vi "Initialize.vi"(8 "error in":errorcluster, 11 "Plugin in":refnum<class "Stereo Microphone Input.lvclass">) -> (0 "error out":errorcluster, 3 "Plugin out":refnum<class "Stereo Microphone Input.lvclass">)   [LabVIEW 2026, in "Stereo Microphone Input.lvlib" / "Stereo Microphone Input.lvclass"]
uses:
  Stereo Microphone Input.lvclass
  C:/Program Files/National Instruments/LabVIEW 2026/vi.lib/FlexLogger/SDK/PluginSDK.lvlibp/PEFClasses/SDK/Plugin/Plugin.lvclass
  <vilib>/FlexLogger/SDK/PluginSDK.lvlibp/PEFClasses/SDK/Processing Element/Timing Parameters.ctl
  <vilib>/FlexLogger/SDK/PluginSDK.lvlibp/PEFClasses/SDK/Processing Element/Timing Method.ctl
  <vilib>/FlexLogger/SDK/PluginSDK.lvlibp/PEFClasses/SDK/Producer Channel/Producer Channel.lvclass
  C:/Program Files/National Instruments/LabVIEW 2026/vi.lib/FlexLogger/SDK/PluginSDK.lvlibp/PEFClasses/SDK/Channel/Channel.lvclass
  <vilib>/FlexLogger/SDK/PluginSDK.lvlibp/PEFClasses/SDK/Plugin/ParameterAccess/Write String.vi
  <vilib>/FlexLogger/SDK/PluginSDK.lvlibp/PEFClasses/SDK/Plugin/ParameterAccess/Write DBL.vi
  <vilib>/FlexLogger/SDK/PluginSDK.lvlibp/PEFClasses/SDK/Producer Channel/Create Producer Channel_v2.vi
  <vilib>/FlexLogger/SDK/PluginSDK.lvlibp/PEFClasses/SDK/Channel/ParameterAccess/Write DBL.vi
  <vilib>/FlexLogger/SDK/PluginSDK.lvlibp/PEFClasses/SDK/Plugin/Plugin.lvclass
  C:/Program Files/National Instruments/LabVIEW 2026/vi.lib/FlexLogger/SDK/PluginSDK.lvlibp/PEFClasses/SDK/Processing Element/Processing Element.lvclass
  C:/Users/nkirchne/Documents/LabVIEW Projects/FlexLogger IO Plug-ins/Stereo Microphone Input/Stereo Microphone Input.lvclass
  C:/Program Files/National Instruments/LabVIEW 2026/vi.lib/FlexLogger/SDK/PluginSDK.lvlibp/PEFClasses/SDK/Producer Channel/Producer Channel.lvclass
  <vilib>/FlexLogger/SDK/PluginSDK.lvlibp/PEFClasses/SDK/Processing Element/Processing Element.lvclass
  <vilib>/FlexLogger/SDK/PluginSDK.lvlibp/PEFClasses/SDK/Channel/Channel.lvclass
  <vilib>/FlexLogger/SDK/PluginSDK.lvlibp
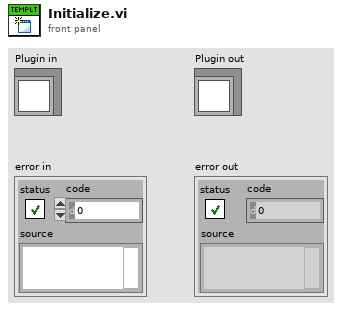
[diagram p1: front panel]
types:
  T1 = typedef "PluginSDK.lvlibp/Processing Element.lvclass/Timing Parameters.ctl" = cluster{"Timing Method":T2, "Timing Period (ms)":i32}
  T2 = typedef "PluginSDK.lvlibp/Processing Element.lvclass/Timing Method.ctl" = enum16{"Periodic", "Immediate", "On Data Ready", "Triggered"}
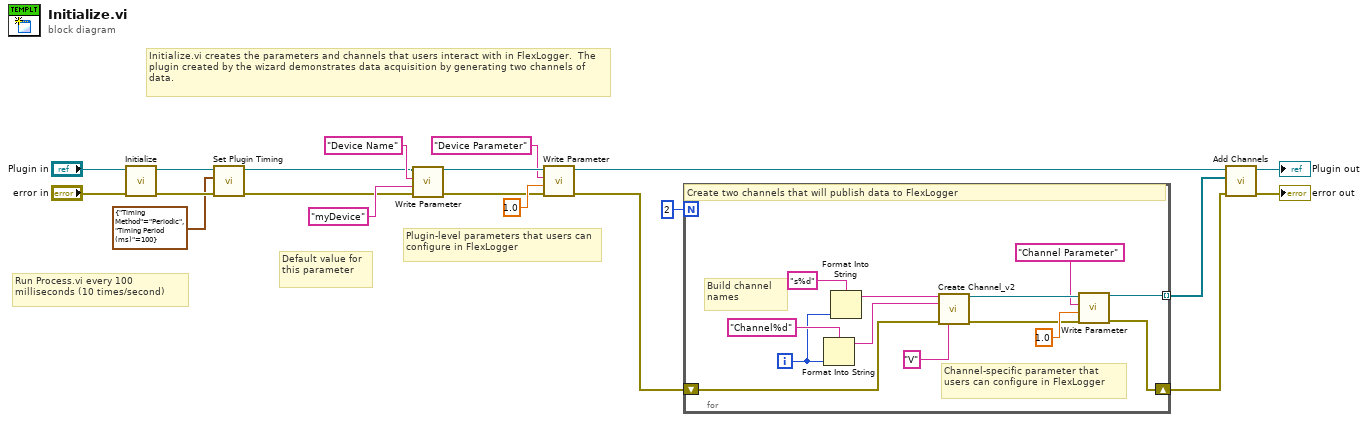
[diagram p0: block diagram]
diagram:
  # "Default value for this parameter"
  # "Plugin-level parameters that users can configure in FlexLogger"
  # "Run Process.vi every 100 milliseconds (10 times/second)"
  # "Initialize.vi creates the parameters and channels that users interact with in FlexLogger.  The plugin created by the wizard demonstrates data acquisition by generating two channels of data."
  n1 = call-parent "Initialize.vi"("error in (no error)"="error in", "Plugin in"="Plugin in") -> ("error out"=w5:errorcluster, "Plugin out"=w3:refnum<class "Stereo Microphone Input.lvclass">)  [unwired: 8 in]
  n2 = call <vilib>:"Set Plugin Timing.vi"("error in (no error)"=w5, "Timing Parameters"=T1 {"Timing Method"=enum."Periodic", "Timing Period (ms)"=100}, "Plugin in"=w3) -> ("error out"=w1:errorcluster, "Plugin out"=w2:refnum<class "Stereo Microphone Input.lvclass">)  [unwired: 7 in]
  n3 = call-poly <vilib>:"Write Parameter.vi"("error in (no error)"=w1, "Value"="myDevice", "Name"="Device Name", "Plugin in"=w2) -> ("error out"=w9:errorcluster, "Plugin out"=w14:refnum<class "Stereo Microphone Input.lvclass">)  [unwired: 6 in]
  n4 = call-poly <vilib>:"Write Parameter.vi"("error in (no error)"=w9, "Value"=1.0, "Name"="Device Parameter", "Plugin in"=w14) -> ("error out"=w8:errorcluster, "Plugin out"=w13:refnum<class "Stereo Microphone Input.lvclass">)  [unwired: 6 in]
  n5 = for {
    N: 2 -> [_]
    shift-right: [w23] -> w15
    shift-left: w8 -> [w22]
    tunnel: [w25] -> w7 mode=indexing
    i -> [w24]
    # "Build channel names"
    # "Channel-specific parameter that users can configure in FlexLogger"
    # "Create two channels that will publish data to FlexLogger"
    n6 = Format Into String(format string="Channel%d", w24) -> (resulting string=w32:string)  [unwired: 2 in, 1 out]
    n7 = Format Into String(format string="s%d", w24) -> (resulting string=w31:string)  [unwired: 2 in, 1 out]
    n8 = call-poly <vilib>:"Create Channel_v2.vi"("Unique Channel Identifier"=w31, "Default Channel Name"=w32, "error in (no error)"=w22, "Unit"="V") -> ("Producer Channel"=w33:refnum<class "Producer Channel.lvclass">, "error out"=w21:errorcluster)  [unwired: 10 in]
    n9 = call-poly <vilib>:"Write Parameter.vi"("error in (no error)"=w21, "Value"=1.0, "Name"="Channel Parameter", "Channel in"=w33) -> ("error out"=w23:errorcluster, "Channel out"=w25:refnum<class "Producer Channel.lvclass">)  [unwired: 6 in]
  }
  n10 = call <vilib>:"Add Channels.vi"("error in (no error)"=w15, "Channels"=w7, "Plugin in"=w13) -> ("error out"=→"error out":errorcluster, "Plugin out"=→"Plugin out":refnum<class "Stereo Microphone Input.lvclass">)  [unwired: 7 in]
